vi "12-1.vi"() -> ()   [LabVIEW 2019, in "12.lvlib"]
uses:
  12.lvlib
  e1706d2a-1850-4533-9028-034c938844d6.vi
panel:
  out "size(s)":i32[](array[numeric])
  out "Routes out":string[][](array[string])
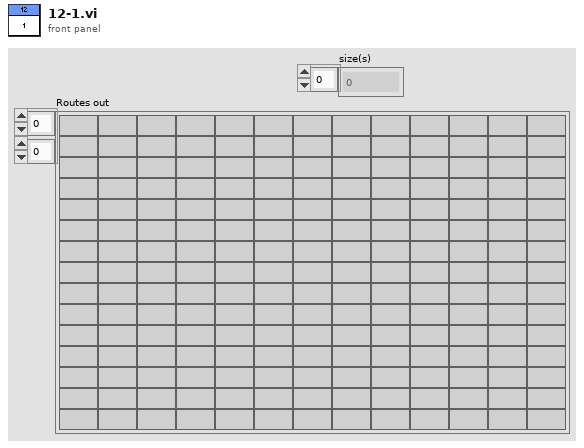
[diagram p1: front panel]
types:
  T1 = cluster{"Cave":string, "Small(F)/Big(T)":bool, "Visited(F)/Not Visited(T)":bool, "Connected Caves":string[]}
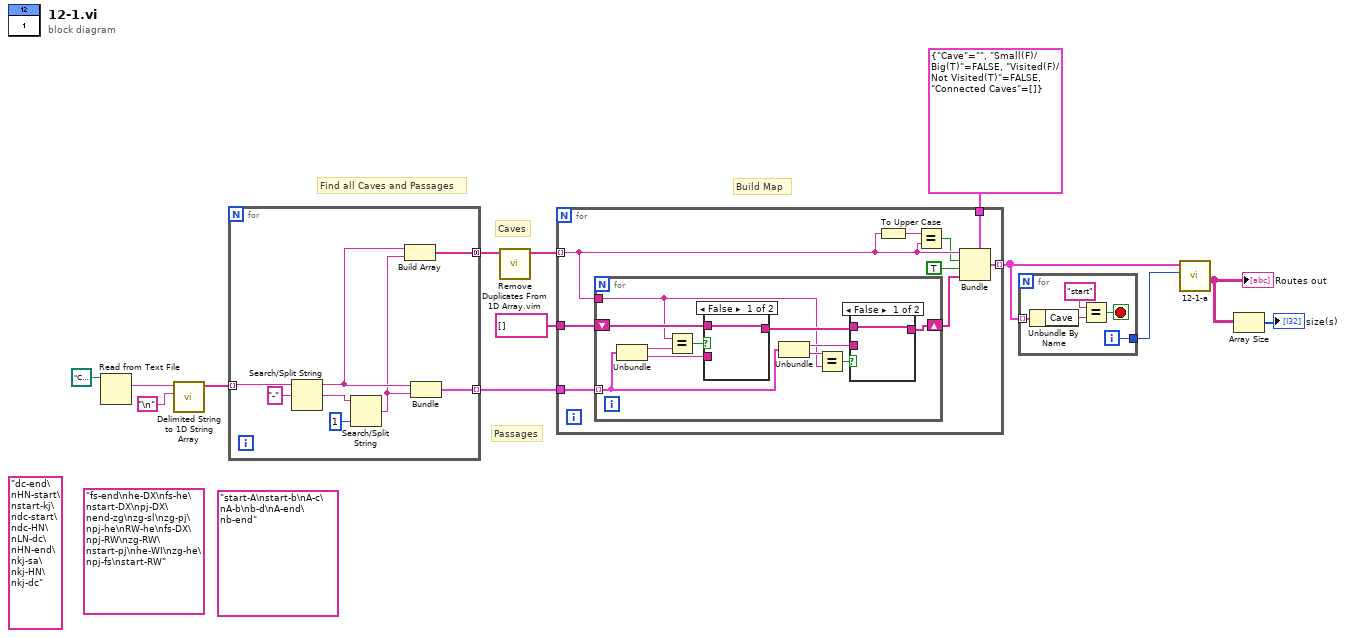
[diagram p0: block diagram]
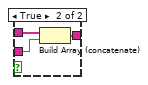
[diagram p2: hidden frame]
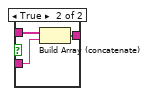
[diagram p3: hidden frame]
diagram:
  (unwired) "fs-end\nhe-DX\nfs-he\nstart-DX\npj-DX\nend-zg\nzg-sl\nzg-pj\npj-he\nRW-he\nfs-DX\npj-RW\nzg-RW\nstart-pj\nhe-WI\nzg-he\npj-fs\nstart-RW"
  (unwired) "dc-end\nHN-start\nstart-kj\ndc-start\ndc-HN\nLN-dc\nHN-end\nkj-sa\nkj-HN\nkj-dc"
  (unwired) "start-A\nstart-b\nA-c\nA-b\nb-d\nA-end\nb-end"
  # "Build Map"
  # "Find all Caves and Passages"
  # "Passages"
  # "Caves"
  n1 = Read from Text File(file (use dialog)=path "C:/Users/craig.walker/Documents/GitHub/lv2019-Advent-of-Code-2021/12/input.txt") -> (text=w2:string)  [unwired: 3 in, 3 out]
  n2 = call <vilib>:"Delimited String to 1D String Array.vi"("delimiter"="\n", "delimited string"=w2) -> ("string array"=w12:string[])  [unwired: 9 in]
  n3 = for {
    tunnel: w12 -> [w21] mode=indexing
    tunnel: [w16] -> w11 mode=concatenating
    tunnel: [w14] -> w9 mode=indexing
    n4 = Search/Split String(string=w21, search string/char (-)="-") -> (substring before match=w19:string, match + rest of string=w18:string)  [unwired: 1 in, 1 out]
    n5 = Search/Split String(string=w18, offset (0)=1) -> (match + rest of string=w15:string)  [unwired: 1 in, 2 out]
    n6 = Build Array(w19, w15) -> (w16:string[])
    n7 = Bundle("String"=w19, "String"=w15) -> (w14:cluster{"String":string, "String":string})  [unwired: 1 in]
  }
  n8 = call "Remove Duplicates From 1D Array.vim"("array"=w11) -> ("array with duplicates removed"=w10:string[])  [unwired: 10 in]
  n9 = for {
    tunnel: w10 -> [w26] mode=indexing
    tunnel: w9 -> [w30]
    tunnel: string[] [] -> [w29]
    tunnel: T1 {"Cave"="", "Small(F)/Big(T)"=FALSE, "Visited(F)/Not Visited(T)"=FALSE, "Connected Caves"=[]} ("cluster") -> [w23]
    tunnel: [w22] -> w5 mode=indexing
    n10 = for {
      tunnel: w30 -> [w32] mode=indexing
      tunnel: w26 -> [w33]
      shift-right: [w31] -> w28
      shift-left: w29 -> [w39]
      n11 = Unbundle(w32) -> ("String"=w40:string, "String"=w38:string)
      n12 = Equal?(x=w33, y=w40) -> (x = y?=w41:bool)
      n13 = case shown="False" w41 {
        tunnel: w39 -> [w46 w49]
        tunnel: w38 -> [_ w48]
        tunnel: [w46 w47] -> w37
        frame False {
        }
        frame True {
          n14 = Build Array (concatenate)(w49, w48) -> (w47:string[])
        }
      }
      n15 = Unbundle(w32) -> ("String"=w35:string, "String"=w34:string)
      n16 = Equal?(x=w34, y=w33) -> (x = y?=w36:bool)
      n17 = case shown="False" w36 {
        tunnel: w37 -> [w42 w45]
        tunnel: w35 -> [_ w44]
        tunnel: [w42 w43] -> w31
        frame False {
        }
        frame True {
          n18 = Build Array (concatenate)(w45, w44) -> (w43:string[])
        }
      }
    }
    n19 = To Upper Case(1:w26) -> (0:w27:string)
    n20 = Equal?(x=w27, y=w26) -> (x = y?=w25:bool)
    n21 = Bundle(cluster=w23, "Cave"=w26, "Small(F)/Big(T)"=w25, "Visited(F)/Not Visited(T)"=TRUE ("x = y?"), "Connected Caves"=w28) -> (w22:T1)
  }
  n22 = for {
    tunnel: w5 -> [w54] mode=indexing
    tunnel: [w50] -> w6
    i -> [w50]
    stop <- w51 stop-if-true
    n23 = Unbundle By Name(w54) -> ("Cave"=w53:string)
    n24 = Equal?(x="start", y=w53) -> (x = y?=w51:bool)
  }
  n25 = call "12-1-a.vi"("Numeric"=w6, "Array"=w5) -> ("Route out"=w4:string[][])  [unwired: 9 in]
  "Routes out" <- w4
  n26 = Array Size(array=w4) -> (size(s)=→"size(s)":i32[])
